vi "ConvertXYMotorDirection.vi"(1 "XY Vector":dbl[](array[numeric])) -> (0 "XY Motor Directions":dbl[](array[numeric]))   [LabVIEW 2015]
uses:
  LabVIEW for ezAFM/LV-PGC 2019-05a/In Progress/ezAFM LabVIEW/NMI coordinates.ctl
panel:
  out "Coordinate System Diagram":T1={"OK"=TRUE}
  # "This is a screenshot from the LabView ezAFM Camera. The numerical values representing the different ezAFM directions are displayed below."
  # "CAD Cartesian Layout"
  # "+x"
  # "+y"
  # "IMAQ Pixel Coordinates"
  # "+x"
  # "0,0"
  # "+y"
  # "ezAFM Coordinates"
  # "+y"
  # "ezAFM coordinates are \nexactly the negative of\nXY values in CAD design"
  # "+x"
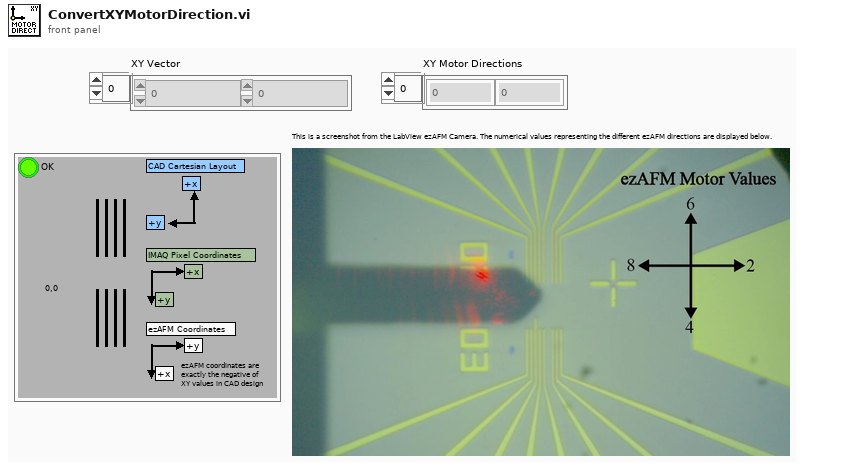
[diagram p1: front panel]
types:
  T1 = typedef "NMI coordinates.ctl" = cluster{"OK":bool}
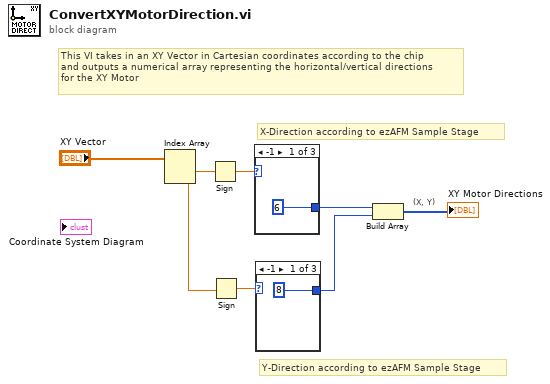
[diagram p0: block diagram]
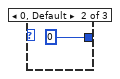
[diagram p2: hidden frame]
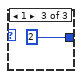
[diagram p3: hidden frame]
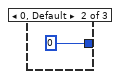
[diagram p4: hidden frame]
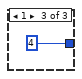
[diagram p5: hidden frame]
diagram:
  # "(X, Y)"
  # "Y-Direction according to ezAFM Sample Stage"
  # "X-Direction according to ezAFM Sample Stage"
  # "This VI takes in an XY Vector in Cartesian coordinates according to the chip\nand outputs a numerical array representing the horizontal/vertical directions\nfor the XY Motor"
  n1 = Index Array(array="XY Vector") -> (element #1=w2:dbl, element #2=w1:dbl)  [unwired: 2 in]
  n2 = Sign(1:w2) -> (0:w7:dbl)
  n3 = Sign(1:w1) -> (0:w6:dbl)
  n4 = case shown="-1" w7 {
    tunnel: [6 0 4] -> w3
    frame -1 {
    }
    frame 0, Default {
    }
    frame 1 {
    }
  }
  n5 = case shown="-1" w6 {
    tunnel: [8 0 2] -> w4
    frame -1 {
    }
    frame 0, Default {
    }
    frame 1 {
    }
  }
  n6 = Build Array(w3, w4) -> (→"XY Motor Directions":i32[])
